vi "CmdSetZeroValue.vi"(8 "error in":errorcluster, 10 "Device Key In":string, 11 "PM Cmds In":refnum<k24>) -> (0 "error out":errorcluster, 1 "I/O Status":i32, 2 "Device Key Out":string, 3 "PM Cmds Out":refnum<k24>)   [LabVIEW 2009]
uses:
  C:/Code/Apps/Utilities/PM2935/PMWinApp/PM_Installer/Master/Samples/1918 - 2936 Family/LabVIEW/LabVIEW 2009/PowerMeterCommands.dll
panel:
  in  "Zero Value":sgl
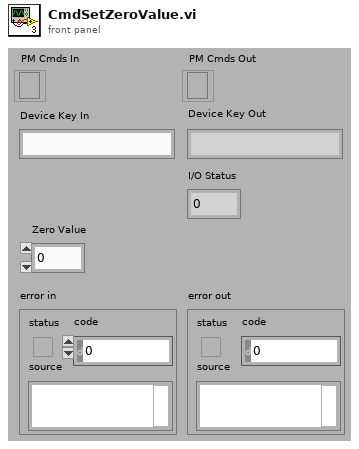
[diagram p1: front panel]
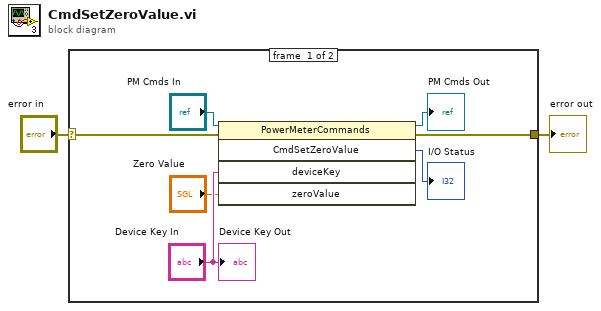
[diagram p0: block diagram]
diagram:
  n1 = case shown="No Error" "error in" {
    selector: "error in" -> [w6 w10]
    tunnel: [w8 w10] -> w2
    frame #0 {
      n2 = invoke class="PowerMeterCommands" method="CmdSetZeroValue"(reference="PM Cmds In", error in=w6, "deviceKey"="Device Key In", "zeroValue"="Zero Value") -> (reference out=→"PM Cmds Out":refnum<k24>, error out=w8:errorcluster, "CmdSetZeroValue"=→"I/O Status":i32)  [unwired: 1 in, 2 out]
      "Device Key Out" <- "Device Key In"
    }
    frame #1 {
    }
  }
  "error out" <- w2
